vi "Relay Tests.vi"(7 "RelayMode":T2, 8 "error in":errorcluster, 9 "Sections":T1, 10 "Socket":i32, 11 "Base path":path=path "C:/Workspace/battery-submodule-eol_oop/Sequence/CodeModules/Hardware Abstraction/Concrete") -> (0 "error out":errorcluster)   [LabVIEW 2019]
uses:
  Controls/RelayMode.ctl
  Config Framework/Controls/Section List.ctl
  Measurment Abstration/MAL.lvlib
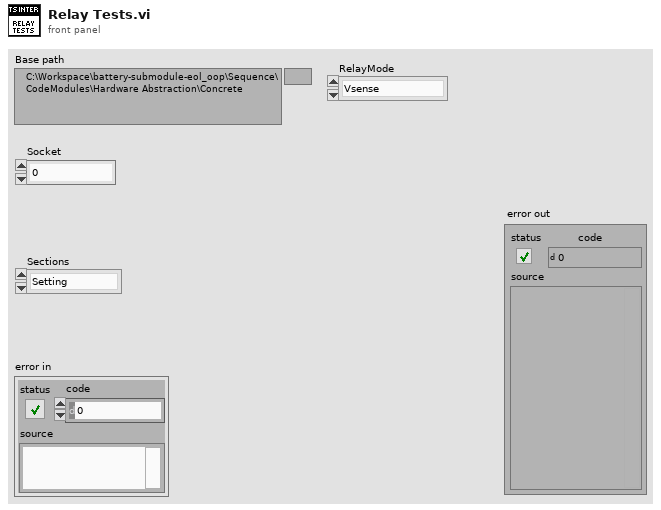
[diagram p1: front panel]
types:
  T1 = typedef "Section List.ctl" = enum16{"Setting", "OPC UA Class Path", "PLC Folder Names", "Ignition Folder Names", "Instruments", "DMM", "ACIR", "HiPOT", "Relay"}
  T2 = typedef "RelayMode.ctl" = enum16{"Vsense", "Thermistor", "ACIR", "HiPOT1", "HiPOT2"}
  T3 = cluster{"Key":string, "Value [1]":string, "Value [2]":string, "Value [3]":string, "Value [4]":string, "Value [5]":string, "Value [6]":string, "Value [7]":string, "Value [8]":string}[]
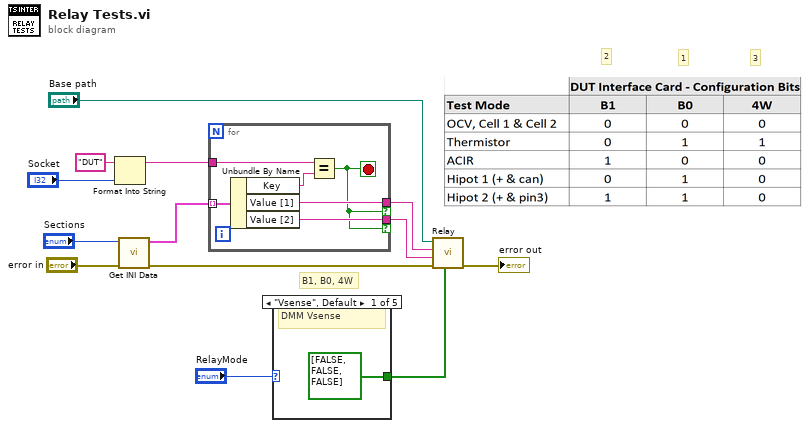
[diagram p0: block diagram]
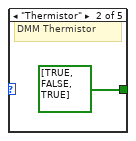
[diagram p2: hidden frame]
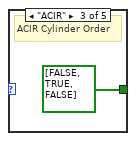
[diagram p3: hidden frame]
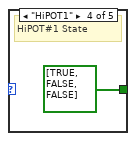
[diagram p4: hidden frame]
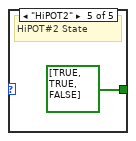
[diagram p5: hidden frame]
diagram:
  # "3"
  # "2"
  # "1"
  # "B1, B0, 4W"
  n1 = Format Into String(initial string="DUT", "Socket") -> (resulting string=w5:string)  [unwired: 2 in, 1 out]
  n2 = call "Get INI Data.vi"("error in"="error in", "Sections"="Sections") -> ("error out"=w9:errorcluster, "INI Data"=w6:T3)  [unwired: 8 in]
  n3 = for {
    tunnel: w6 -> [w17] mode=indexing
    tunnel: w5 -> [w19]
    tunnel: [w16] -> w4 if=w14
    tunnel: [w15] -> w3 if=w14
    stop <- w14 stop-if-true
    n4 = Unbundle By Name(w17) -> ("Key"=w18:string, "Value [1]"=w16:string, "Value [2]"=w15:string)
    n5 = Equal?(x=w19, y=w18) -> (x = y?=w14:bool)
  }
  n6 = case shown="\"Vsense\", Default" "RelayMode" {
    tunnel: [bool[] [FALSE, FALSE, FALSE] bool[] [TRUE, FALSE, TRUE] bool[] [FALSE, TRUE, FALSE] bool[] [TRUE, FALSE, FALSE] bool[] [TRUE, TRUE, FALSE]] -> w10
    frame "Vsense", Default {
      # "DMM Vsense"
    }
    frame "Thermistor" {
      # "DMM Thermistor"
    }
    frame "ACIR" {
      # "ACIR Cylinder Order"
    }
    frame "HiPOT1" {
      # "HiPOT#1 State"
    }
    frame "HiPOT2" {
      # "HiPOT#2 State"
    }
  }
  n7 = call "Relay.vi"("Relay Mode"=w10, "error in"=w9, "Relay Class"=w3, "Line(s)"=w4, "Base Path"="Base path") -> ("error out"=→"error out":errorcluster)  [unwired: 6 in]
